vi "Draw ViewFinder Sign.vi"(9 "Color":u32(colorbox), 11 "2D Picture":picture) -> (3 "2D Picture out":picture)   [LabVIEW 2015]
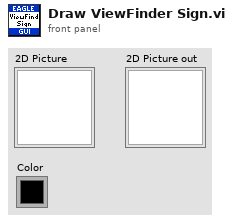
[diagram p1: front panel]
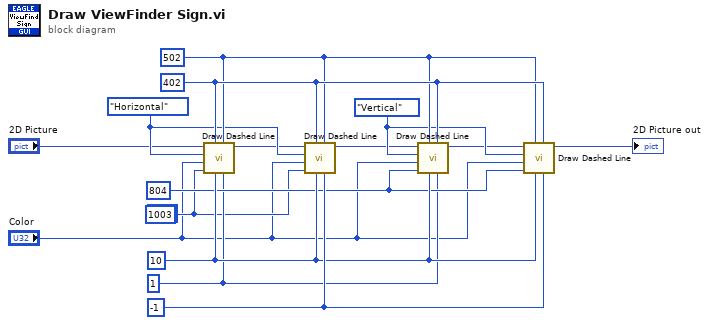
[diagram p0: block diagram]
diagram:
  w9 = enum16{"Horizontal", "Vertical"}."Vertical" ("Type")
  w10 = 804 ("Dimension")
  (unwired) 1003 ("Dimension")
  w13 = 502 ("Dynamic Origin")
  w14 = 402 ("Static Origin")
  w12 = -1 ("Direction")
  w7 = 1 ("Direction")
  w11 = 10 ("Line Width")
  w5 = 1003 ("Dimension")
  w4 = enum16{"Horizontal", "Vertical"}."Horizontal" ("Type")
  n1 = call "Draw Dashed Line.vi"("Direction"=w7, "Dynamic Origin"=w13, "Line Width"=w11, "Static Origin"=w14, "Dimension"=w5, "Color"="Color", "Type"=w4, "2D Picture in"="2D Picture") -> ("2D Picture out"=w3:picture)  [unwired: 3 in]
  n2 = call "Draw Dashed Line.vi"("Direction"=w12, "Dynamic Origin"=w13, "Line Width"=w11, "Static Origin"=w14, "Dimension"=w5, "Color"="Color", "Type"=w4, "2D Picture in"=w3) -> ("2D Picture out"=w6:picture)  [unwired: 3 in]
  n3 = call "Draw Dashed Line.vi"("Direction"=w7, "Dynamic Origin"=w14, "Line Width"=w11, "Static Origin"=w13, "Dimension"=w10, "Color"="Color", "Type"=w9, "2D Picture in"=w6) -> ("2D Picture out"=w8:picture)  [unwired: 3 in]
  n4 = call "Draw Dashed Line.vi"("Direction"=w12, "Dynamic Origin"=w14, "Line Width"=w11, "Static Origin"=w13, "Dimension"=w10, "Color"="Color", "Type"=w9, "2D Picture in"=w8) -> ("2D Picture out"=→"2D Picture out":picture)  [unwired: 3 in]
